vi "初始设置.vi"(0 "引用句柄输入":refnum<k21>, 5 "error out":errorcluster caption="错误输出") -> (12 "就绪状态":bool=TRUE, 14 "task out":refnum<k21>, 19 "error IO":errorcluster)   [LabVIEW 2018]
uses:
  <vilib>/DAQmx/create/channels.llb/DAQmx Create Channel (AI-Sound Pressure-Microphone).vi
  <vilib>/DAQmx/configure/timing.llb/DAQmx Timing (Sample Clock).vi
  <resource>/objmgr/daqmx.rc
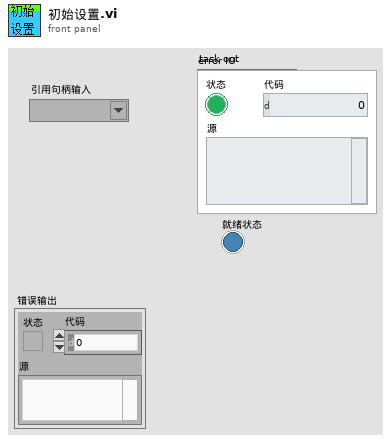
[diagram p1: front panel]
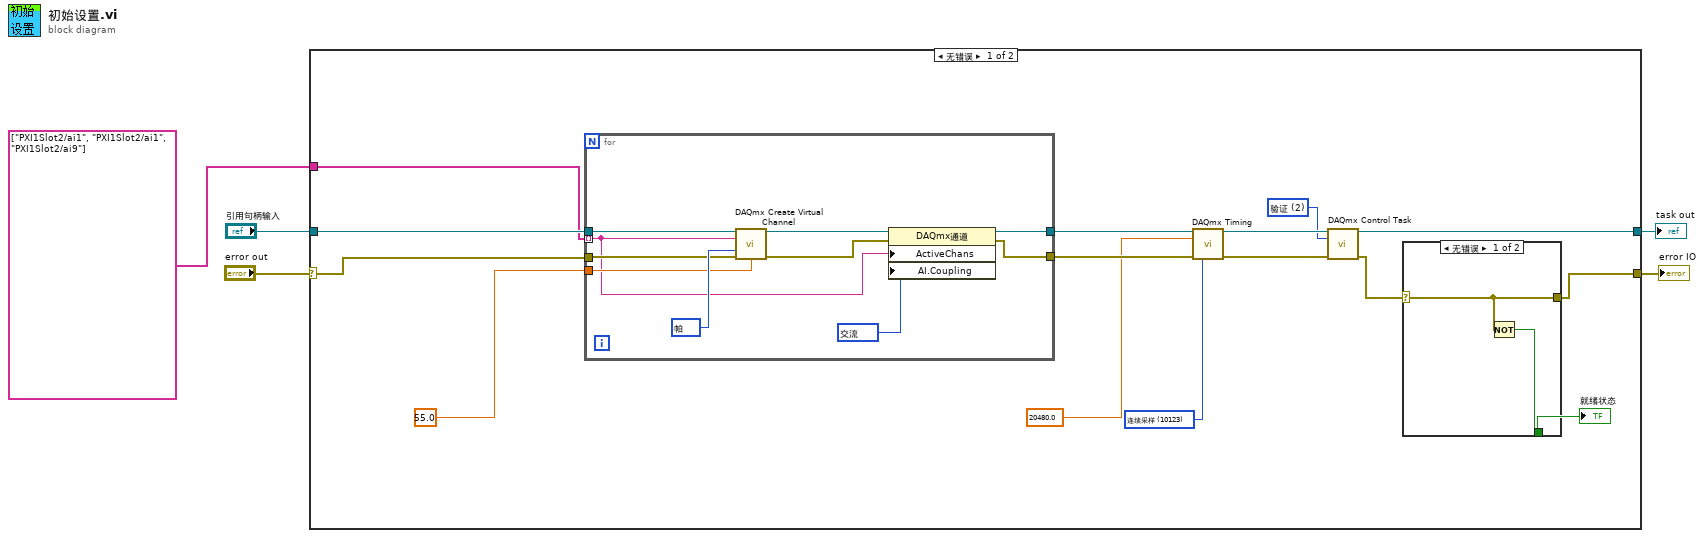
[diagram p0: block diagram]
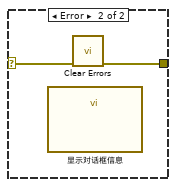
[diagram p2: hidden frame]
diagram:
  n1 = case shown="无错误" "error out" {
    selector: "error out" -> [w19 w36]
    tunnel: "引用句柄输入" -> [w20 w35]
    tunnel: [w13 w35] -> w4
    tunnel: [w8 w36] -> w2
    tunnel: tag[] ["PXI1Slot2/ai1", "PXI1Slot2/ai1", "PXI1Slot2/ai9"] ("physical channels") -> [w7 _]
    frame No Error {
      w11 = 2 items=["验证"=2, "保留"=4, "提交"=3, "未保留"=5, "中止"=6] ("action")
      w15 = 10123 items=["有限采样"=10178, "连续采样"=10123, "硬件定时单点"=12522] ("sample mode")
      n2 = for {
        tunnel: w7 -> [w25] mode=indexing
        tunnel: w20 -> [w33]
        tunnel: 55.0 -> [w32]
        tunnel: [w29] -> w18
        tunnel: [w27] -> w17
        tunnel: w19 -> [w31]
        w26 = 10045 items=["交流"=10045, "直流"=10050, "GND"=10066] ("AI.Coupling")
        w34 = 10081 items=["帕"=10081, "来自自定义换算"=10065] ("units")
        n3 = call-poly <vilib>:"DAQmx Create Virtual Channel.vi"("task in"=w33, "physical channels"=w25, "units"=w34, "error in"=w31, "microphone sensitivity"=w32) -> ("task out"=w30:refnum<k21>, "error out"=w28:errorcluster)  [unwired: 9 in]
        n4 = property class="DAQmx通道"(reference=w30, error in=w28, "ActiveChans"=w25, "AI.Coupling"=w26) -> (reference out=w29:refnum<k21>, error out=w27:errorcluster)
      }
      n5 = call-poly <vilib>:"DAQmx Timing.vi"("task/channels in"=w18, "sample mode"=w15, "rate"=20480.0, "error in"=w17) -> ("task out"=w14:refnum<k21>, "error out"=w12:errorcluster)  [unwired: 10 in]
      n6 = call <vilib>:"DAQmx Control Task.vi"("task/channels in"=w14, "action"=w11, "error in"=w12) -> ("task out"=w13:refnum<k21>, "error out"=w10:errorcluster)  [unwired: 11 in]
      n7 = case shown="无错误" w10 {
        selector: w10 -> [w21 w24]
        tunnel: [w22 _] -> w9
        tunnel: [w21 w23] -> w8
        frame No Error {
          n8 = Not(x=w21) -> (.not. x?=w22:bool)
        }
        frame Error {
          n9 = call "显示对话框信息"() -> ()  [unwired: 10 in, 2 out]
          n10 = call <vilib>:"Clear Errors.vi"("error in (no error)"=w24) -> ("error out"=w23:errorcluster)  [unwired: 5 in, 1 out]
        }
      }
      "就绪状态" <- w9
    }
    frame Error {
    }
  }
  "task out" <- w4
  "error IO" <- w2
